vi "Finish.vi"(6 "Sender":refnum<class "Sender.lvclass">, 9 "Error":errorcluster, 10 "Actor":refnum<class "Actor.lvclass">, 11 "Finish in":refnum<class "Finish.lvclass">) -> (0 "Error out":errorcluster, 3 "Finish out":refnum<class "Finish.lvclass">)   [LabVIEW 2025, in "jettl.lvlib" / "Finish Msg.lvlib" / "Finish.lvclass"]
uses:
  Finish.lvclass
  Actor/Actor/Actor.lvclass
  Sender/Sender/Sender.lvclass
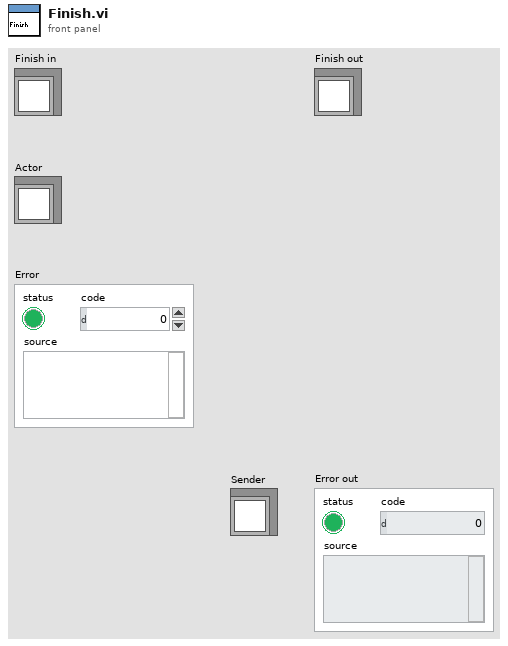
[diagram p1: front panel]
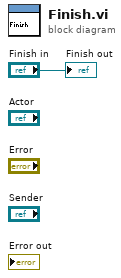
[diagram p0: block diagram]
diagram:
  "Finish out" <- "Finish in"
